vi "Get Rx Monitor All Channels Array.vi"() -> (1 "channel array":string[](array[string]))   [LabVIEW 2020, in "AIM ARINC 664 Scripting.lvlib"]
uses:
  AIM ARINC 664 Scripting.lvlib
  Constants.vi
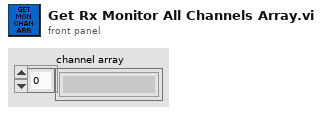
[diagram p1: front panel]
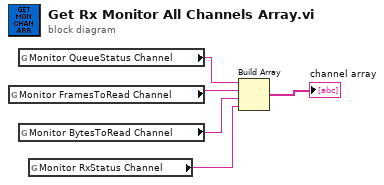
[diagram p0: block diagram]
diagram:
  n1 = global read "Constants.vi" "Monitor FramesToRead Channel"() -> (w5:string)
  n2 = global read "Constants.vi" "Monitor QueueStatus Channel"() -> (w3:string)
  n3 = global read "Constants.vi" "Monitor BytesToRead Channel"() -> (w4:string)
  n4 = global read "Constants.vi" "Monitor RxStatus Channel"() -> (w1:string)
  n5 = Build Array(w3, w5, w4, w1) -> (→"channel array":string[])
